vi "replaceVIWithItemFromNewLibrary.vi"(6 "SubVI Path":path, 8 "error in (no error)":errorcluster, 9 "SubVI Refnum":refnum<vi>, 10 "Calling VI Reference":refnum<vi>, 11 "Dependency in":refnum<class "Dependency.lvclass">) -> (0 "error out":errorcluster, 3 "Dependency out":refnum<class "Dependency.lvclass">)   [LabVIEW 2016, in "Dependency.lvclass"]
uses:
  Dependency.lvclass
  Dependency.lvclass/Dependency.ctl
  Search/Search.lvclass/Search.ctl
  Variables/VIsReplaced.vi
  Variables/VIsReplaceFailed.vi
  Search/Search.lvclass
  Variables/SwitchDependenciesVariables.lvlib
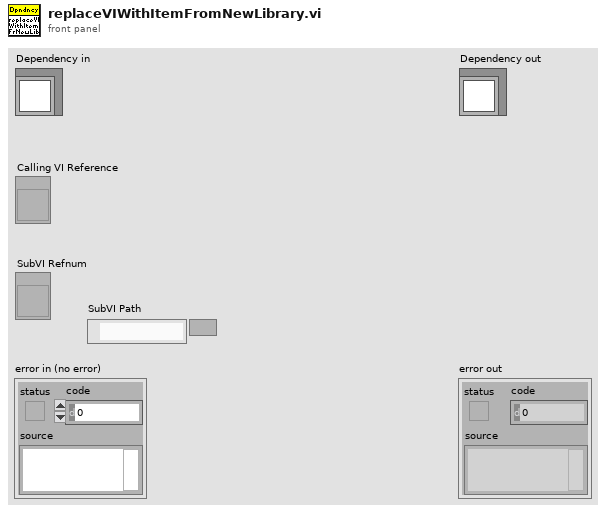
[diagram p1: front panel]
types:
  T1 = typedef "LibraryMemberNameReplacement.ctl" = cluster{"String To Replace in VI names":string, "String To Replace in Control names":string, "New String in VI names":string, "New String in Control names":string}
  T2 = typedef "LibraryDirectories.ctl" = cluster{"OldLibraryDirectory":string, "NewLibraryDirectory":string}
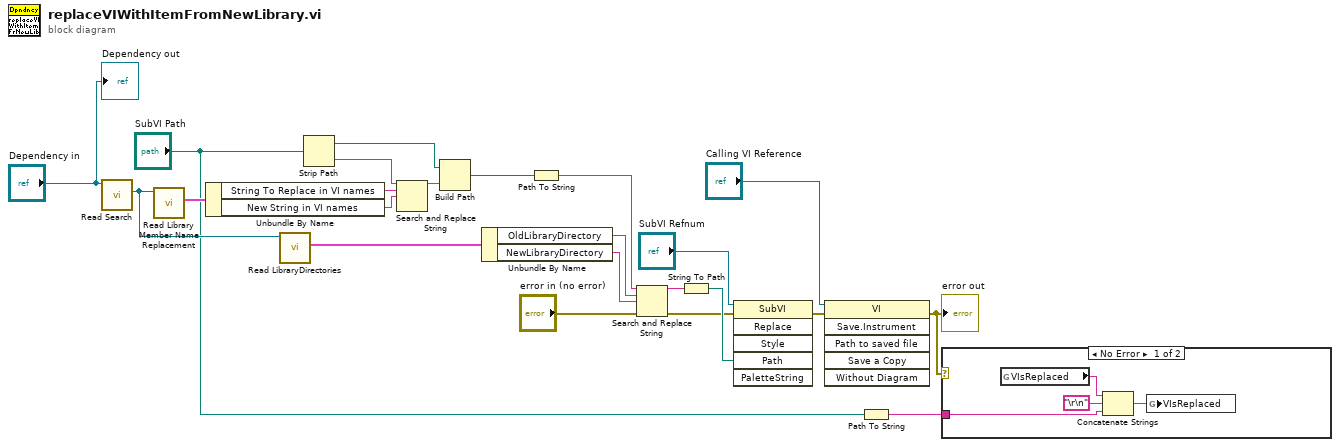
[diagram p0: block diagram]
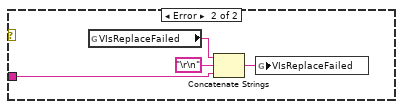
[diagram p2: hidden frame]
diagram:
  n1 = call "Read Search.vi"("Dependency in"="Dependency in") -> ("Search"=w7:refnum<class "Search.lvclass">)  [unwired: 9 in, 1 out]
  n2 = call "Read Library Member Name Replacement.vi"("ProjectItem in"=w7) -> ("Library Member Name Replacement"=w6:T1)  [unwired: 9 in, 1 out]
  n3 = Unbundle By Name(w6) -> ("String To Replace in VI names"=w18:string, "New String in VI names"=w17:string)
  n4 = call "Read LibraryDirectories.vi"("ProjectItem in"=w7) -> ("LibraryDirectories"=w8:T2)  [unwired: 9 in, 1 out]
  n5 = Strip Path(path="SubVI Path") -> (stripped path=w16:path, name=w19:string)
  n6 = Search and Replace String(input string=w19, search string=w18, replace string=w17) -> (result string=w15:string)  [unwired: 5 in, 3 out]
  n7 = Build Path(base path=w16, name or relative path=w15) -> (appended path=w14:path)
  n8 = Unbundle By Name(w8) -> ("OldLibraryDirectory"=w11:string, "NewLibraryDirectory"=w10:string)
  n9 = Path To String(path=w14) -> (string=w13:string)
  n10 = Search and Replace String(input string=w13, search string=w11, replace string=w10, error in="error in (no error)") -> (result string=w12:string, error out=w1:errorcluster)  [unwired: 4 in, 2 out]
  n11 = String To Path(string=w12) -> (path=w23:path)
  n12 = invoke class="SubVI" method="Replace"(reference="SubVI Refnum", error in=w1, "Path"=w23) -> (error out=w21:errorcluster)  [unwired: 3 in, 5 out]
  n13 = invoke class="VI" method="Save.Instrument"(reference="Calling VI Reference", error in=w21) -> (error out=w4:errorcluster)  [unwired: 4 in, 5 out]
  "error out" <- w4
  n14 = Path To String(path="SubVI Path") -> (string=w5:string)
  n15 = case shown="No Error" w4 {
    tunnel: w5 -> [w25 w29]
    frame No Error {
      n16 = global read "VIsReplaced.vi" "VIsReplaced"() -> (w27:string)
      n17 = Concatenate Strings(w27, "\r\n", w25) -> (w24:string)
      n18 = global write "VIsReplaced.vi" "VIsReplaced"(w24) -> ()
    }
    frame Error {
      n19 = global read "VIsReplaceFailed.vi" "VIsReplaceFailed"() -> (w31:string)
      n20 = Concatenate Strings(w31, "\r\n", w29) -> (w28:string)
      n21 = global write "VIsReplaceFailed.vi" "VIsReplaceFailed"(w28) -> ()
    }
  }
  "Dependency out" <- "Dependency in"
